vi "Vacum Valve Control.vi"(8 "error in":errorcluster, 11 "HTS Results in":refnum<class "HTS Results.lvclass">) -> (0 "error out":errorcluster, 1 "Valve Pos":dbl, 2 "Vavum Valve CMD":string="s", 3 "HTS Results out":refnum<class "HTS Results.lvclass">)   [LabVIEW 2019, in "Results.lvlib" / "HTS Results.lvclass"]
uses:
  HTS Results.lvclass
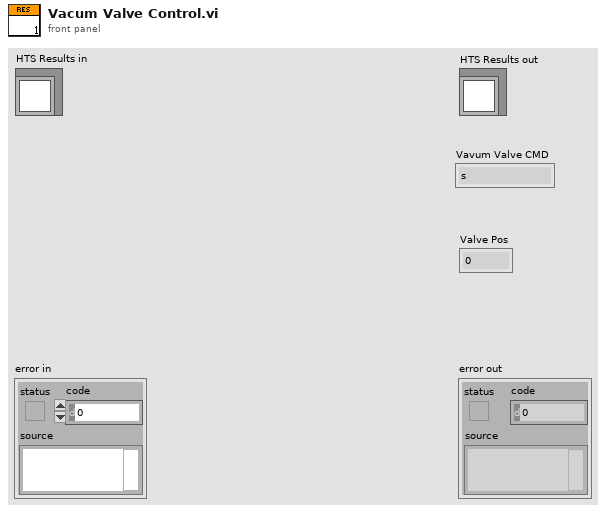
[diagram p1: front panel]
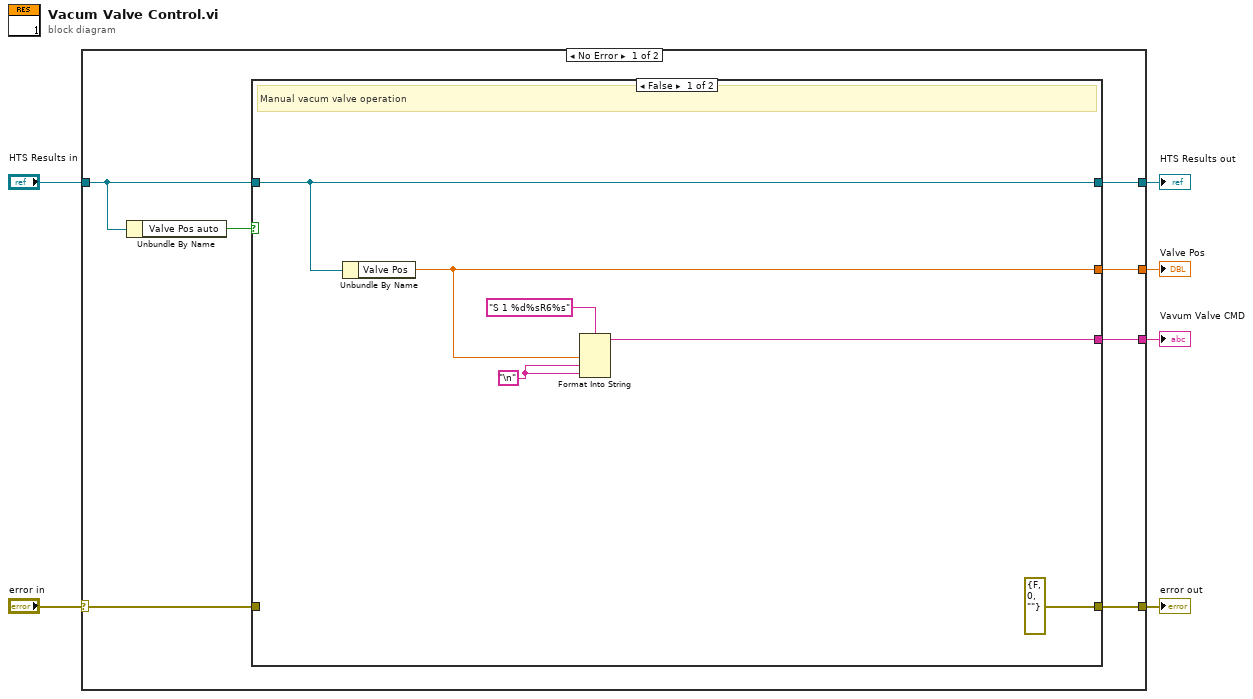
[diagram p0: block diagram]
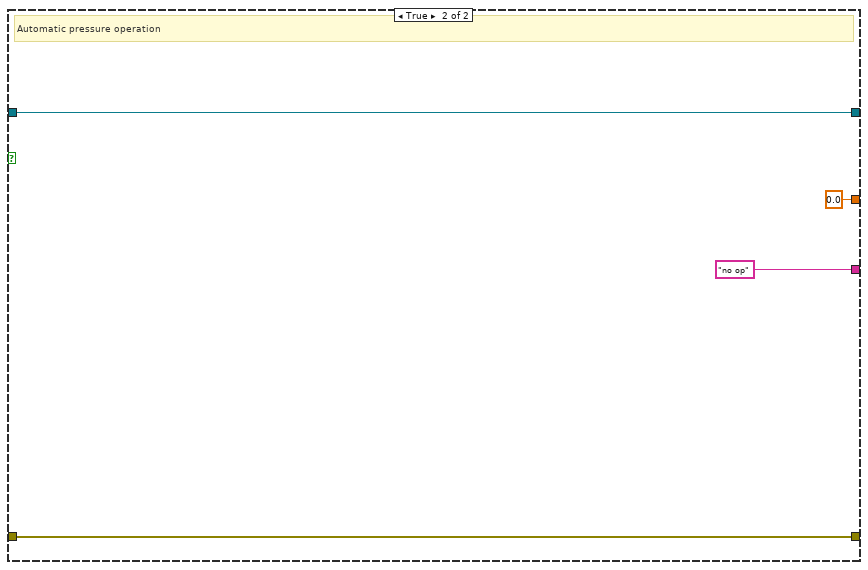
[diagram p2: hidden frame]
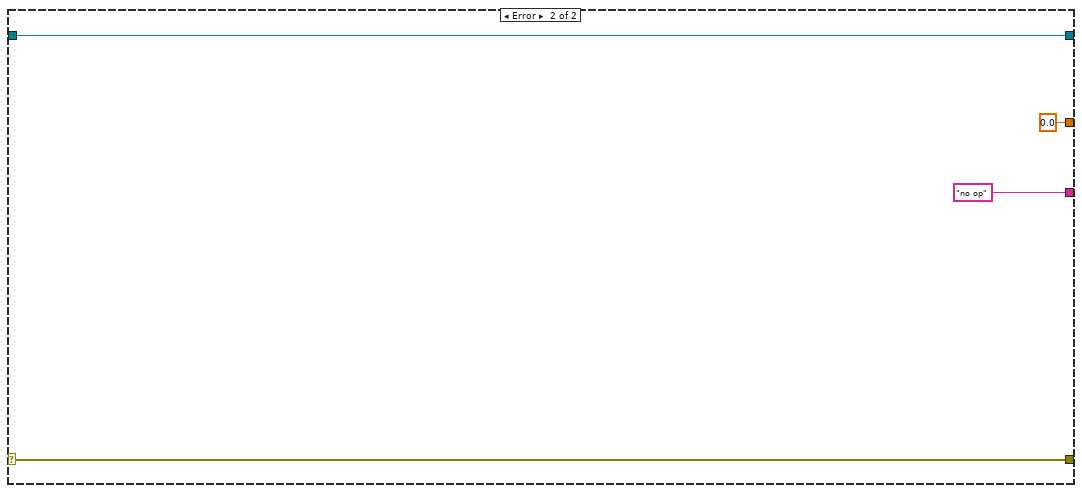
[diagram p3: hidden frame]
diagram:
  n1 = case shown="No Error" "error in" {
    selector: "error in" -> [w8 w27]
    tunnel: [w13 w27] -> w5
    tunnel: "HTS Results in" -> [w12 w26]
    tunnel: [w10 w26] -> w3
    tunnel: [w9 "no op"] -> w2
    tunnel: [w7 0.0 ("Valve Pos")] -> w1
    frame No Error {
      n2 = Unbundle By Name(w12) -> ("Valve Pos auto"=w11:bool)
      n3 = case shown="False" w11 {
        tunnel: [errorcluster {"status"=FALSE, "code"=0, "source"=""} ("error IO") w21] -> w13
        tunnel: w12 -> [w18 w23]
        tunnel: [w18 w23] -> w10
        tunnel: [w15 "no op"] -> w9
        tunnel: w8 -> [_ w21]
        tunnel: [w16 0.0 ("Valve Pos")] -> w7
        frame False {
          w14 = "\n"
          # "Manual vacum valve operation"
          n4 = Unbundle By Name(w18) -> ("Valve Pos"=w16:dbl)
          n5 = Format Into String(format string="S 1 %d%sR6%s", w16, w14, w14) -> (resulting string=w15:string)  [unwired: 2 in, 1 out]
        }
        frame True {
          # "Automatic pressure operation"
        }
      }
    }
    frame Error {
    }
  }
  "error out" <- w5
  "HTS Results out" <- w3
  "Vavum Valve CMD" <- w2
  "Valve Pos" <- w1
